vi "PXI-Handle Device Specific Gains.vi"(0 "AO Tasks in":T1[](array[typedef]), 11 "error in (no error)":errorcluster) -> (4 "AO Tasks out":T1[](array[typedef]), 15 "error out":errorcluster)   [LabVIEW 2020]
uses:
  Type Defs/Task Struct.ctl
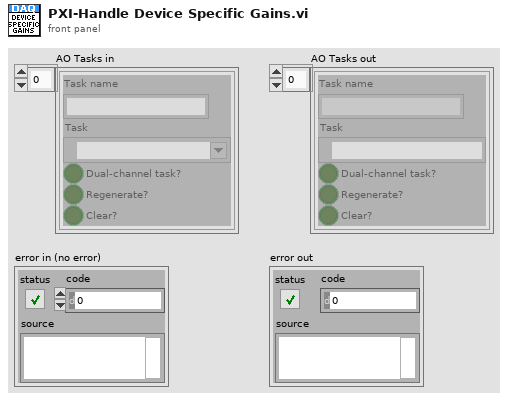
[diagram p1: front panel]
types:
  T1 = typedef "Task Struct.ctl" = cluster{"Task name":string, "Task":refnum<k21>, "Dual-channel task?":bool, "Regenerate?":bool, "Clear?":bool}
  T2 = enum16{"Init", "Write", "Read", "Latch setup", "Compute comp.", "Read 1 Channel"}
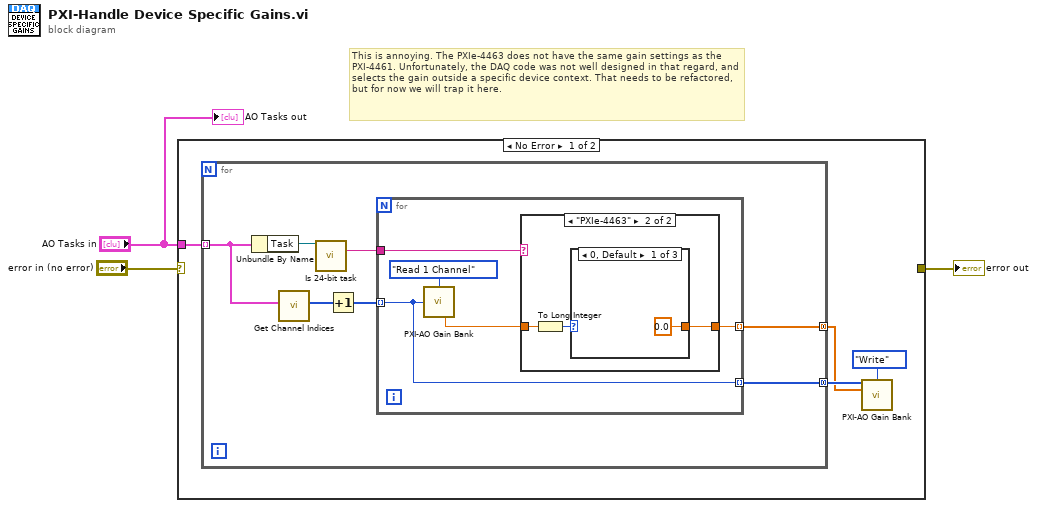
[diagram p0: block diagram]
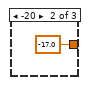
[diagram p3: hidden frame]
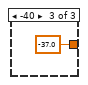
[diagram p4: hidden frame]
diagram:
  # "This is annoying. The PXIe-4463 does not have the same gain settings as the PXI-4461. Unfortunately, the DAQ code was not well designed in that regard, and selects the gain outside a specific device context. That needs to be refactored, but for now we will trap it here."
  n1 = case shown="No Error" "error in (no error)" {
    selector: "error in (no error)" -> [_ w27]
    tunnel: "AO Tasks in" -> [w7 _]
    tunnel: [_ w27] -> w1
    frame No Error {
      n2 = for {
        tunnel: w7 -> [w13] mode=indexing
        tunnel: [w9] -> w4 mode=concatenating
        tunnel: [w8] -> w5 mode=concatenating
        n3 = Unbundle By Name(w13) -> ("Task"=w14:refnum<k21>)
        n4 = call "Get Channel Indices.vi"("Task Structure"=w13) -> ("Channel Indices"=w12:i32[])  [unwired: 10 in]
        n5 = call "Is 24-bit task.vi"("task"=w14) -> ("Product Type"=w10:string)  [unwired: 9 in, 5 out]
        n6 = Increment(x=w12) -> (x+1=w11:i32[])
        n7 = for {
          tunnel: w11 -> [w15] mode=indexing
          tunnel: w10 -> [w18]
          tunnel: [w16] -> w9 mode=indexing
          tunnel: [w15] -> w8 mode=indexing
          n8 = call "PXI-AO Gain Bank.vi"("Action"=T2."Read 1 Channel", "AO channel"=w15) -> ("Gain 1 channel"=w17:dbl)  [unwired: 8 in, 5 out]
          n9 = case shown="\"PXIe-4463\"" w18 {
            tunnel: w17 -> [w20 w23]
            tunnel: [w20 w21] -> w16
            frame "", Default {
            }
            frame "PXIe-4463" {
              n10 = To Long Integer(number=w23) -> (32bit integer=w22:i32)
              n11 = case shown="0, Default" w22 {
                tunnel: [0.0 -17.0 -37.0] -> w21
                frame 0, Default {
                }
                frame -20 {
                }
                frame -40 {
                }
              }
            }
          }
        }
      }
      n12 = call "PXI-AO Gain Bank.vi"("AO Channels"=w5, "Action"=T2."Write", "Gains"=w4) -> ()  [unwired: 7 in, 6 out]
    }
    frame Error {
    }
  }
  "error out" <- w1
  "AO Tasks out" <- "AO Tasks in"
